vi "Bridge serial.vi"() -> ()   [LabVIEW 2018]
uses:
  <vilib>/Instr/_visa.llb/VISA Configure Serial Port (Instr).vi
  Global_Telescopio.vi
panel:
  out "respTUBO":string
  out "cmdTUBO":string
  out "respCUP":string
  out "cmdCUP":string
  out "cmdDEC":string
  out "respDEC":string
  out "respAH":string
  out "cmdAH":string
  in  "stop":bool
  # "Bridge Serial   TCSPD  < -- > Controladores"
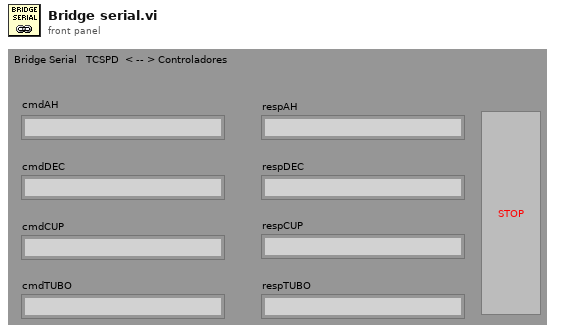
[diagram p1: front panel]
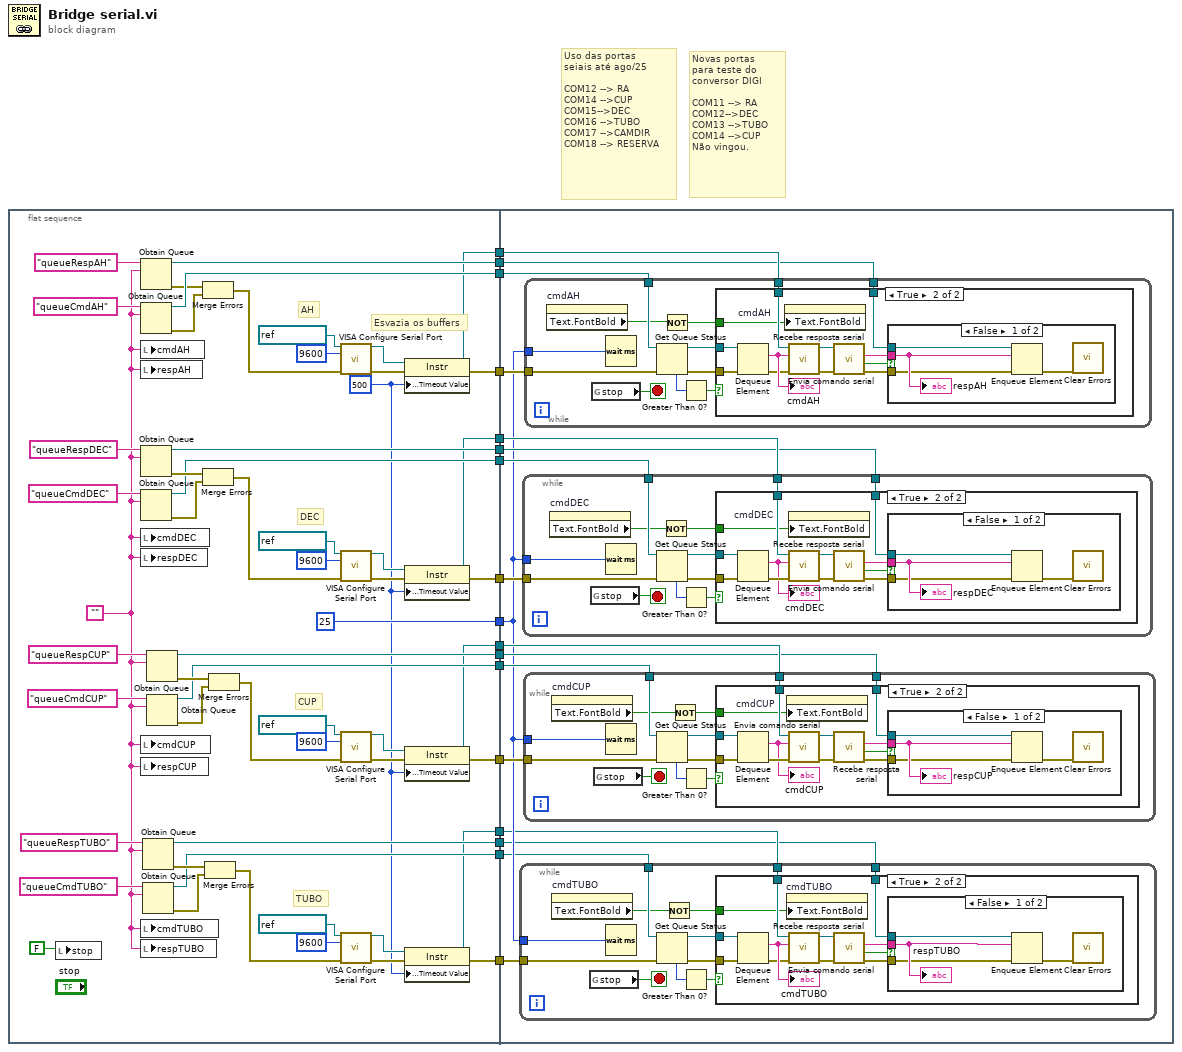
[diagram p0: block diagram]
diagram:
  # "Novas portas\npara teste do\nconversor DIGI\n\nCOM11 --> RA\nCOM12-->DEC\nCOM13 -->TUBO\nCOM14 -->CUP\nNão vingou."
  # "Uso das portas \nseiais até ago/25\n\nCOM12 --> RA\nCOM14 -->CUP\nCOM15-->DEC\nCOM16 -->TUBO\nCOM17 -->CAMDIR\nCOM18 --> RESERVA"
  n1 = flat-sequence {
    tunnel: [w23] -> w17
    tunnel: [w22] -> w16
    tunnel: [w20] -> w15
    tunnel: [w63] -> w14
    tunnel: [w62] -> w13
    tunnel: [w55] -> w12
    tunnel: [w54] -> w11
    tunnel: [u32 25 ("milliseconds to wait")] -> w10
    tunnel: [w46] -> w9
    tunnel: [w45] -> w8
    tunnel: [w40] -> w7
    tunnel: [w38] -> w6
    tunnel: [w33] -> w5
    tunnel: [w31] -> w4
    tunnel: [w25] -> w3
    tunnel: [w21] -> w2
    tunnel: [w24] -> w1
    tunnel: w17 -> [w90]
    tunnel: w16 -> [w89]
    tunnel: w15 -> [w87]
    tunnel: w14 -> [w84]
    tunnel: w13 -> [w86]
    tunnel: w12 -> [w81]
    tunnel: w11 -> [w83]
    tunnel: w10 -> [w77]
    tunnel: w9 -> [w78]
    tunnel: w8 -> [w80]
    tunnel: w7 -> [w74]
    tunnel: w6 -> [w76]
    tunnel: w5 -> [w85]
    tunnel: w4 -> [w82]
    tunnel: w3 -> [w75]
    tunnel: w2 -> [w88]
    tunnel: w1 -> [w79]
    frame #0 {
      w18 = u32 500 ("Tmo Value")
      w39 = ""
      # "Esvazia os buffers"
      # "TUBO"
      # "DEC"
      # "CUP"
      # "AH"
      n2 = local write "stop"(FALSE) -> ()
      n3 = Obtain Queue(name (unnamed)="queueRespAH", element data type=w39) -> (queue out=w63:refnum<queue>, error out=w61:errorcluster)  [unwired: 3 in, 1 out]
      n4 = Obtain Queue(name (unnamed)="queueCmdAH", element data type=w39) -> (queue out=w62:refnum<queue>, error out=w60:errorcluster)  [unwired: 3 in, 1 out]
      n5 = local write "cmdAH"(w39) -> ()
      n6 = local write "respAH"(w39) -> ()
      n7 = Obtain Queue(name (unnamed)="queueRespDEC", element data type=w39) -> (queue out=w55:refnum<queue>, error out=w58:errorcluster)  [unwired: 3 in, 1 out]
      n8 = Obtain Queue(name (unnamed)="queueCmdDEC", element data type=w39) -> (queue out=w54:refnum<queue>, error out=w52:errorcluster)  [unwired: 3 in, 1 out]
      n9 = local write "cmdDEC"(w39) -> ()
      n10 = local write "respDEC"(w39) -> ()
      n11 = local write "cmdCUP"(w39) -> ()
      n12 = local write "respCUP"(w39) -> ()
      n13 = local write "cmdTUBO"(w39) -> ()
      n14 = local write "respTUBO"(w39) -> ()
      n15 = Obtain Queue(name (unnamed)="queueRespTUBO", element data type=w39) -> (queue out=w40:refnum<queue>, error out=w44:errorcluster)  [unwired: 3 in, 1 out]
      n16 = Obtain Queue(name (unnamed)="queueCmdTUBO", element data type=w39) -> (queue out=w38:refnum<queue>, error out=w41:errorcluster)  [unwired: 3 in, 1 out]
      n17 = Obtain Queue(name (unnamed)="queueRespCUP", element data type=w39) -> (queue out=w46:refnum<queue>, error out=w47:errorcluster)  [unwired: 3 in, 1 out]
      n18 = Obtain Queue(name (unnamed)="queueCmdCUP", element data type=w39) -> (queue out=w45:refnum<queue>, error out=w50:errorcluster)  [unwired: 3 in, 1 out]
      n19 = Merge Errors(w61, w60) -> (w59:errorcluster)
      n20 = Merge Errors(w58, w52) -> (w51:errorcluster)
      n21 = Merge Errors(w44, w41) -> (w36:errorcluster)
      n22 = Merge Errors(w47, w50) -> (w37:errorcluster)
      n23 = call-poly "VISA Configure Serial Port"("VISA resource name"=refnum<visa-resource-name> "COM12", "baud rate (9600)"=u32 9600, "error in (no error)"=w59) -> ("VISA resource name out"=w34:refnum<visa-resource-name>, "error out"=w35:errorcluster)  [unwired: 11 in]
      n24 = call-poly "VISA Configure Serial Port"("VISA resource name"=refnum<visa-resource-name> "COM15", "baud rate (9600)"=u32 9600, "error in (no error)"=w51) -> ("VISA resource name out"=w30:refnum<visa-resource-name>, "error out"=w32:errorcluster)  [unwired: 11 in]
      n25 = call-poly "VISA Configure Serial Port"("VISA resource name"=refnum<visa-resource-name> "COM14", "baud rate (9600)"=u32 9600, "error in (no error)"=w37) -> ("VISA resource name out"=w29:refnum<visa-resource-name>, "error out"=w28:errorcluster)  [unwired: 11 in]
      n26 = call-poly "VISA Configure Serial Port"("VISA resource name"=refnum<visa-resource-name> "COM16", "baud rate (9600)"=u32 9600, "error in (no error)"=w36) -> ("VISA resource name out"=w27:refnum<visa-resource-name>, "error out"=w26:errorcluster)  [unwired: 11 in]
      n27 = property class="Instr"(reference=w34, error in=w35, "General Settings:Timeout Value"=w18) -> (reference out=w33:refnum<visa-resource-name>, error out=w23:errorcluster)
      n28 = property class="Instr"(reference=w30, error in=w32, "General Settings:Timeout Value"=w18) -> (reference out=w31:refnum<visa-resource-name>, error out=w22:errorcluster)
      n29 = property class="Instr"(reference=w29, error in=w28, "General Settings:Timeout Value"=w18) -> (reference out=w24:refnum<visa-resource-name>, error out=w21:errorcluster)
      n30 = property class="Instr"(reference=w27, error in=w26, "General Settings:Timeout Value"=w18) -> (reference out=w25:refnum<visa-resource-name>, error out=w20:errorcluster)
    }
    frame #1 {
      n31 = while {
        tunnel: w87 -> [w98]
        tunnel: w77 -> [w97]
        tunnel: w76 -> [w96]
        tunnel: w75 -> [w95]
        tunnel: w74 -> [w94]
        stop <- w93 stop-if-true
        n32 = property on="cmdTUBO" class="Str"() -> ("Text.FontBold"=w92:bool)  [unwired: 2 in, 2 out]
        n33 = global read "Global_Telescopio.vi" "stop"() -> (w93:bool)
        n34 = Wait (ms)(milliseconds to wait=w97) -> ()  [unwired: 1 out]
        n35 = Get Queue Status(queue=w96, error in (no error)=w98) -> (queue out=w100:refnum<queue>, error out=w99:errorcluster, # elements in queue=w102:i32)  [unwired: 1 in, 5 out]
        n36 = Not(x=w92) -> (.not. x?=w91:bool)
        n37 = Greater Than 0?(x=w102) -> (x > 0?=w101:bool)
        n38 = case shown="True" w101 {
          tunnel: w100 -> [_ w114]
          tunnel: w99 -> [_ w106]
          tunnel: w95 -> [_ w105]
          tunnel: w94 -> [_ w104]
          tunnel: w91 -> [_ w103]
          frame False {
          }
          frame True {
            n39 = Dequeue Element(queue=w114, error in (no error)=w106) -> (element=w109:string, error out=w107:errorcluster)  [unwired: 1 in, 2 out]
            "cmdTUBO" <- w109
            n40 = property on="cmdTUBO" class="Str"("Text.FontBold"=w103) -> ()  [unwired: 2 in, 2 out]
            n41 = call "Envia comando serial.vi"("error In"=w107, "String a ser Enviado"=w109, "LNA VISA session (for class)"=w105) -> ("error out"=w112:errorcluster, "LNA VISA session saida"=w113:refnum<visa-resource-name>)  [unwired: 2 in, 1 out]
            n42 = call "Recebe resposta serial.vi"("error in (no error)"=w112, "LNA VISA resource name"=w113) -> ("error out"=w108:errorcluster, "timeout"=w111:bool, "String Lida"=w110:string)  [unwired: 6 in, 1 out]
            n43 = case shown="False" w111 {
              tunnel: w110 -> [w118 _]
              tunnel: w108 -> [w116 _]
              tunnel: w104 -> [w115 _]
              frame False {
                n44 = Enqueue Element(queue=w115, element=w118, error in (no error)=w116) -> (error out=w117:errorcluster)  [unwired: 1 in, 2 out]
                n45 = call <vilib>:"Clear Errors.vi"("error in (no error)"=w117) -> ()  [unwired: 5 in, 2 out]
                "respTUBO" <- w118
              }
              frame True {
              }
            }
          }
        }
      }
      n46 = while {
        tunnel: w89 -> [w154]
        tunnel: w83 -> [w153]
        tunnel: w82 -> [w152]
        tunnel: w81 -> [w151]
        tunnel: w77 -> [w150]
        stop <- w149 stop-if-true
        n47 = property on="cmdDEC" class="Str"() -> ("Text.FontBold"=w148:bool)  [unwired: 2 in, 2 out]
        n48 = global read "Global_Telescopio.vi" "stop"() -> (w149:bool)
        n49 = Wait (ms)(milliseconds to wait=w150) -> ()  [unwired: 1 out]
        n50 = Get Queue Status(queue=w153, error in (no error)=w154) -> (queue out=w156:refnum<queue>, error out=w155:errorcluster, # elements in queue=w158:i32)  [unwired: 1 in, 5 out]
        n51 = Not(x=w148) -> (.not. x?=w147:bool)
        n52 = Greater Than 0?(x=w158) -> (x > 0?=w157:bool)
        n53 = case shown="True" w157 {
          tunnel: w156 -> [_ w170]
          tunnel: w155 -> [_ w163]
          tunnel: w152 -> [_ w161]
          tunnel: w151 -> [_ w160]
          tunnel: w147 -> [_ w159]
          frame False {
          }
          frame True {
            n54 = Dequeue Element(queue=w170, error in (no error)=w163) -> (element=w162:string, error out=w164:errorcluster)  [unwired: 1 in, 2 out]
            "cmdDEC" <- w162
            n55 = property on="cmdDEC" class="Str"("Text.FontBold"=w159) -> ()  [unwired: 2 in, 2 out]
            n56 = call "Envia comando serial.vi"("error In"=w164, "String a ser Enviado"=w162, "LNA VISA session (for class)"=w161) -> ("error out"=w168:errorcluster, "LNA VISA session saida"=w169:refnum<visa-resource-name>)  [unwired: 2 in, 1 out]
            n57 = call "Recebe resposta serial.vi"("error in (no error)"=w168, "LNA VISA resource name"=w169) -> ("error out"=w165:errorcluster, "timeout"=w167:bool, "String Lida"=w166:string)  [unwired: 6 in, 1 out]
            n58 = case shown="False" w167 {
              tunnel: w166 -> [w174 _]
              tunnel: w165 -> [w172 _]
              tunnel: w160 -> [w171 _]
              frame False {
                n59 = Enqueue Element(queue=w171, element=w174, error in (no error)=w172) -> (error out=w173:errorcluster)  [unwired: 1 in, 2 out]
                n60 = call <vilib>:"Clear Errors.vi"("error in (no error)"=w173) -> ()  [unwired: 5 in, 2 out]
                "respDEC" <- w174
              }
              frame True {
              }
            }
          }
        }
      }
      n61 = while {
        tunnel: w88 -> [w126]
        tunnel: w77 -> [w125]
        tunnel: w80 -> [w124]
        tunnel: w79 -> [w123]
        tunnel: w78 -> [w122]
        stop <- w121 stop-if-true
        n62 = property on="cmdCUP" class="Str"() -> ("Text.FontBold"=w120:bool)  [unwired: 2 in, 2 out]
        n63 = global read "Global_Telescopio.vi" "stop"() -> (w121:bool)
        n64 = Wait (ms)(milliseconds to wait=w125) -> ()  [unwired: 1 out]
        n65 = Get Queue Status(queue=w124, error in (no error)=w126) -> (queue out=w128:refnum<queue>, error out=w127:errorcluster, # elements in queue=w130:i32)  [unwired: 1 in, 5 out]
        n66 = Not(x=w120) -> (.not. x?=w119:bool)
        n67 = Greater Than 0?(x=w130) -> (x > 0?=w129:bool)
        n68 = case shown="True" w129 {
          tunnel: w128 -> [_ w142]
          tunnel: w127 -> [_ w135]
          tunnel: w123 -> [_ w134]
          tunnel: w122 -> [_ w133]
          tunnel: w119 -> [_ w131]
          frame False {
          }
          frame True {
            n69 = Dequeue Element(queue=w142, error in (no error)=w135) -> (element=w132:string, error out=w136:errorcluster)  [unwired: 1 in, 2 out]
            "cmdCUP" <- w132
            n70 = property on="cmdCUP" class="Str"("Text.FontBold"=w131) -> ()  [unwired: 2 in, 2 out]
            n71 = call "Envia comando serial.vi"("error In"=w136, "String a ser Enviado"=w132, "LNA VISA session (for class)"=w134) -> ("error out"=w140:errorcluster, "LNA VISA session saida"=w141:refnum<visa-resource-name>)  [unwired: 2 in, 1 out]
            n72 = call "Recebe resposta serial.vi"("error in (no error)"=w140, "LNA VISA resource name"=w141) -> ("error out"=w137:errorcluster, "timeout"=w139:bool, "String Lida"=w138:string)  [unwired: 6 in, 1 out]
            n73 = case shown="False" w139 {
              tunnel: w138 -> [w146 _]
              tunnel: w137 -> [w144 _]
              tunnel: w133 -> [w143 _]
              frame False {
                n74 = Enqueue Element(queue=w143, element=w146, error in (no error)=w144) -> (error out=w145:errorcluster)  [unwired: 1 in, 2 out]
                n75 = call <vilib>:"Clear Errors.vi"("error in (no error)"=w145) -> ()  [unwired: 5 in, 2 out]
                "respCUP" <- w146
              }
              frame True {
              }
            }
          }
        }
      }
      n76 = while {
        tunnel: w90 -> [w183]
        tunnel: w86 -> [w181]
        tunnel: w85 -> [w180]
        tunnel: w84 -> [w179]
        tunnel: w77 -> [w178]
        stop <- w177 stop-if-true
        n77 = property on="cmdAH" class="Str"() -> ("Text.FontBold"=w176:bool)  [unwired: 2 in, 2 out]
        n78 = global read "Global_Telescopio.vi" "stop"() -> (w177:bool)
        n79 = Wait (ms)(milliseconds to wait=w178) -> ()  [unwired: 1 out]
        n80 = Get Queue Status(queue=w181, error in (no error)=w183) -> (queue out=w184:refnum<queue>, error out=w182:errorcluster, # elements in queue=w186:i32)  [unwired: 1 in, 5 out]
        n81 = Not(x=w176) -> (.not. x?=w175:bool)
        n82 = Greater Than 0?(x=w186) -> (x > 0?=w185:bool)
        n83 = case shown="True" w185 {
          tunnel: w184 -> [_ w198]
          tunnel: w182 -> [_ w192]
          tunnel: w180 -> [_ w189]
          tunnel: w179 -> [_ w188]
          tunnel: w175 -> [_ w187]
          frame False {
          }
          frame True {
            n84 = Dequeue Element(queue=w198, error in (no error)=w192) -> (element=w193:string, error out=w191:errorcluster)  [unwired: 1 in, 2 out]
            "cmdAH" <- w193
            n85 = property on="cmdAH" class="Str"("Text.FontBold"=w187) -> ()  [unwired: 2 in, 2 out]
            n86 = call "Envia comando serial.vi"("error In"=w191, "String a ser Enviado"=w193, "LNA VISA session (for class)"=w189) -> ("error out"=w196:errorcluster, "LNA VISA session saida"=w197:refnum<visa-resource-name>)  [unwired: 2 in, 1 out]
            n87 = call "Recebe resposta serial.vi"("error in (no error)"=w196, "LNA VISA resource name"=w197) -> ("error out"=w190:errorcluster, "timeout"=w195:bool, "String Lida"=w194:string)  [unwired: 6 in, 1 out]
            n88 = case shown="False" w195 {
              tunnel: w194 -> [w202 _]
              tunnel: w190 -> [w201 _]
              tunnel: w188 -> [w199 _]
              frame False {
                n89 = Enqueue Element(queue=w199, element=w202, error in (no error)=w201) -> (error out=w200:errorcluster)  [unwired: 1 in, 2 out]
                n90 = call <vilib>:"Clear Errors.vi"("error in (no error)"=w200) -> ()  [unwired: 5 in, 2 out]
                "respAH" <- w202
              }
              frame True {
              }
            }
          }
        }
      }
    }
  }
